vi "table line to assembly.vi"(11 "ItemNames":string[](array[string])) -> (3 "assembly definition":T1)   [LabVIEW 2013, in "EthernetIP editor node.lvclass"]
uses:
  EthernetIP editor node.lvclass
  <vilib>/NI/TBM Modules/Ethernet IP/configuration/assembly definition.ctl
  <vilib>/NI/TBM Modules/Ethernet IP/configuration/assembly type.ctl
  <vilib>/NI/TBM Modules/Ethernet IP/configuration/EthernetIP configuration.lvclass
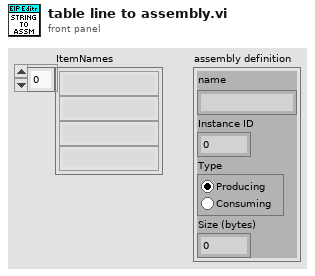
[diagram p1: front panel]
types:
  T1 = typedef "EthernetIP configuration.lvclass/assembly definition.ctl" = cluster{"name":string, "Instance ID":u32, "Type":T2, "Size (bytes)":u32}
  T2 = typedef "EthernetIP configuration.lvclass/assembly type.ctl" = enum32{"Producing", "Consuming"}
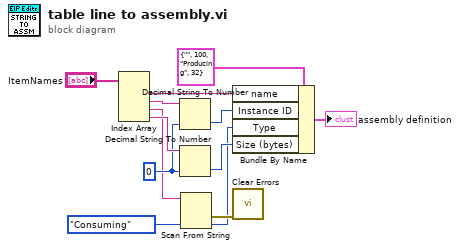
[diagram p0: block diagram]
diagram:
  w5 = u32 0 ("default (0 I32)")
  n1 = Index Array(array="ItemNames") -> (element #1=w10:string, element #2=w9:string, element #3=w1:string, element #4=w8:string)  [unwired: 4 in]
  n2 = Decimal String To Number(string=w9, default (0L)=w5) -> (number=w6:u32)  [unwired: 1 in, 1 out]
  n3 = Decimal String To Number(string=w8, default (0L)=w5) -> (number=w7:u32)  [unwired: 1 in, 1 out]
  n4 = Scan From String(input string=w1, default 1=assembly_type."Consuming" ("Type")) -> (error out=w4:errorcluster, output 1=w3:T2)  [unwired: 3 in, 2 out]
  n5 = Bundle By Name(cluster=T1 {"name"="", "Instance ID"=100, "Type"=enum."Producing", "Size (bytes)"=32} ("assembly definition"), "name"=w10, "Instance ID"=w6, "Type"=w3, "Size (bytes)"=w7) -> (→"assembly definition":T1)
  n6 = call <vilib>:"Clear Errors.vi"("error in (no error)"=w4) -> ()  [unwired: 6 in, 1 out]
